vi "Write permissions.vi"(8 "error in (no error)":errorcluster, 10 "permissions":u32 format="%04o", 11 "file attributes in":refnum<class "File Attributes.lvclass">) -> (0 "error out":errorcluster, 3 "file attributes out":refnum<class "File Attributes.lvclass">)   [LabVIEW 2020, in "NI_SFTP.lvlib" / "File Attributes.lvclass"]
doc: "Writes Unix numeric permissions information into this File Attributes object. Use this property with <b>Set File Attributes</b> to update the permissions of a remote file or directory."
uses:
  <vilib>/net/SFTP/File Attributes/File Attributes.lvclass
  <vilib>/net/SFTP/File Attributes/File Attributes.lvclass/File Attributes.ctl
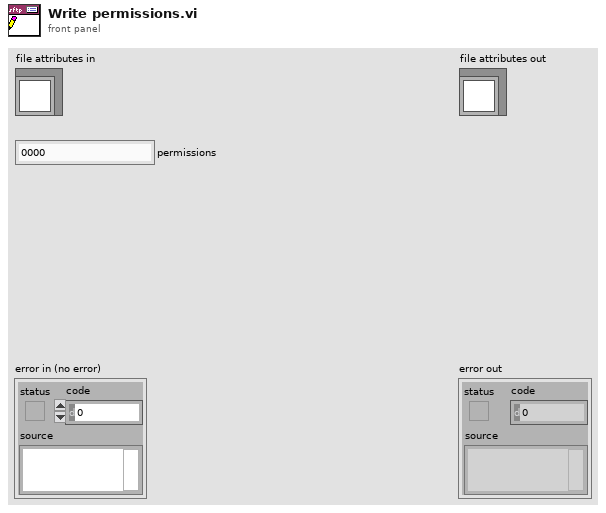
[diagram p1: front panel]
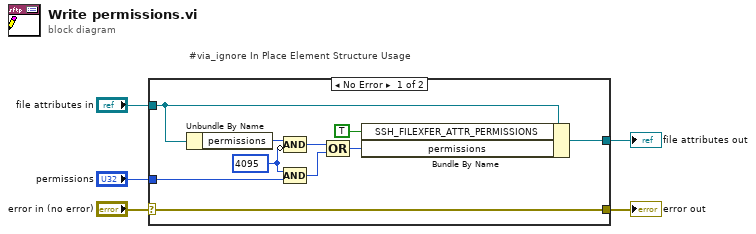
[diagram p0: block diagram]
diagram:
  # "#via_ignore In Place Element Structure Usage"
  n1 = case shown="No Error" "error in (no error)" {
    selector: "error in (no error)" -> [w15 w16]
    tunnel: [w15 w16] -> w4
    tunnel: [w14 w17] -> w2
    tunnel: "file attributes in" -> [w12 w17]
    tunnel: "permissions" -> [w10 _]
    frame No Error {
      w9 = u32 4095
      n2 = Unbundle By Name(w12) -> ("permissions"=w11:u32)
      n3 = Compound Arithmetic op=AND(w11, invert w9) -> (w8:u32)
      n4 = Compound Arithmetic op=AND(w9, w10) -> (w7:u32)
      n5 = Compound Arithmetic op=OR(w8, w7) -> (w6:u32)
      n6 = Bundle By Name(cluster=w12, "SSH_FILEXFER_ATTR_PERMISSIONS"=TRUE ("SFTP Session.lvclass:Name.File Attributes.SSH_FILEXFER_ATTR_PERMISSIONS"), "permissions"=w6) -> (w14:refnum<class "File Attributes.lvclass">)
    }
    frame Error {
    }
  }
  "error out" <- w4
  "file attributes out" <- w2
